vi "MixingGUI_ManyMixtures_OLD.vi"() -> ()   [LabVIEW 2016]
uses:
  <vilib>/Utility/miscctls.llb/LVStringsAndValuesArrayTypeDef.ctl
  <userlib>/Fluigent/Fluigent MFCS/FluigentMFCS_Full.llb/MFCS_EZ Detect.vi
  <userlib>/Fluigent/Fluigent MFCS/FluigentMFCS_Full.llb/MFCS_EZ Initialization.vi
  <userlib>/Fluigent/Fluigent MFCS/FluigentMFCS_Full.llb/MFCS_EZ Write Channel Pressure.vi
  Globals/PressuresGlobal.vi
  Labjack/ValveGlobals.vi
  <vilib>/Utility/file.llb/Write Delimited Spreadsheet (string).vi
  <vilib>/Utility/file.llb/Read Delimited Spreadsheet (string).vi
  <userlib>/_OpenG.lib/array/array.llb/Remove Duplicates from 1D Array (U16)__ogtk.vi
  <vilib>/Utility/xml.llb/Read From XML File(string).vi
  <vilib>/Utility/xml.llb/Write to XML File(string).vi
  <userlib>/Fluigent/Fluigent MFCS/FluigentMFCS_Full.llb/MFCS_EZ Close.vi
  <vilib>/MakerHub/Toolbox/LMH-Toolbox.lvlib
panel:
  out "Set Pressure Cluster":T1={"Control Pressure"=291.6495768427234, "Set Water Mix Pressures"=[nan, nan, nan, nan, nan, 1003.8886388678504, 1033.3198159146239, nan, 1065.755981313159], "Set Odor Pressures"=[nan, nan, 914.431476155127, 919.4749175766236]}
  out "Possible Water Mix Ratios":dbl[](array[numeric])=[0.1, 0.2, 0.30000000000000004, 0.4, 0.5, 0.6, 0.7, 0.7999999999999999, 0.8999999999999999]
  in  "Begin Experiment":bool
  out "Log Folder":path=path "E:/maggot images/Jacob/20180701"
  in  "Master Timing":dbl[][](array[numeric])=[[10.0, 10.0, 10.0], [10.0, 10.0, 10.0]]
  in  "Number of Periods":u16=3
  in  "Master Mix Cluster":T2(array[cluster])=[{"Edit Mixture"=FALSE, "Mixture List"="1.0E-6 1-pentanol", "Odor Time"=10.0, "Water Time"=10.0, "Number of Odors"=1}, {"Edit Mixture"=FALSE, "Mixture List"="1.0E-6 1-pentanol", "Odor Time"=10.0, "Water Time"=10.0, "Number of Odors"=1}, {"Edit Mixture"=FALSE, "Mixture List"="", "Odor Time"=10.0, "Water Time"=10.0, "Number of Odors"=0}, {"Edit Mixture"=FALSE, "Mixture List"="1.0E-7 2,5-dimethylthiazole", "Odor Time"=10.0, "Water Time"=10.0, "Number of Odors"=1}, {"Edit Mixture"=FALSE, "Mixture List"="1.0E-6 acetal", "Odor Time"=10.0, "Water Time"=10.0, "Number of Odors"=1}, {"Edit Mixture"=FALSE, "Mixture List"="1.0E-6 2-phenyl ethanol", "Odor Time"=10.0, "Water Time"=10.0, "Number of Odors"=1}, {"Edit Mixture"=FALSE, "Mixture List"="1.0E-7 2-methoxyphenyl acetate", "Odor Time"=10.0, "Water Time"=10.0, "Number of Odors"=1}, {"Edit Mixture"=FALSE, "Mixture List"="1.0E-7 4-methyl-5-vinythiazole", "Odor Time"=10.0, "Water Time"=10.0, "Number of Odors"=1}, {"Edit Mixture"=FALSE, "Mixture List"="1.0E-6 1-pentanol", "Odor Time"=10.0, "Water Time"=10.0, "Number of Odors"=1}, {"Edit Mixture"=FALSE, "Mixture List"="1.0E-6 1-pentanol\r1.0E-7 4-methyl-5-vinythiazole", "Odor Time"=10.0, "Water Time"=10.0, "Number of Odors"=2}, {"Edit Mixture"=FALSE, "Mixture List"="", "Odor Time"=10.0, "Water Time"=10.0, "Number of Odors"=0}, {"Edit Mixture"=FALSE, "Mixture List"="", "Odor Time"=10.0, "Water Time"=10.0, "Number of Odors"=0}, {"Edit Mixture"=FALSE, "Mixture List"="", "Odor Time"=10.0, "Water Time"=8.0, "Number of Odors"=0}, {"Edit Mixture"=FALSE, "Mixture List"="", "Odor Time"=10.0, "Water Time"=10.0, "Number of Odors"=0}, {"Edit Mixture"=FALSE, "Mixture List"="", "Odor Time"=10.0, "Water Time"=10.0, "Number of Odors"=0}, {"Edit Mixture"=FALSE, "Mixture List"="", "Odor Time"=10.0, "Water Time"=10.0, "Number of Odors"=0}, {"Edit Mixture"=FALSE, "Mixture List"="", "Odor Time"=10.0, "Water Time"=10.0, "Number of Odors"=0}, {"Edit Mixture"=FALSE, "Mixture List"="", "Odor Time"=10.0, "Water Time"=10.0, "Number of Odors"=0}]
  out "Odor Strings":string[](array[string])=["1-pentanol", "3-pentanol", "3-octanol", "2,5-dimethylthiazole", "acetal", "2-phenyl ethanol", "2-methoxyphenyl acetate", "4-methyl-5-vinythiazole"]
  out "Concentration Strings":string[](array[string])=["1.0E-6", "1.0E-7", "1.0E-7", "1.0E-7", "1.0E-6", "1.0E-6", "1.0E-7", "1.0E-7"]
  out "Master Mix Sequence Array":bool[][](array[boolean])=[[TRUE, FALSE, FALSE, FALSE, FALSE, FALSE, FALSE, FALSE], [TRUE, TRUE, TRUE, FALSE, FALSE, FALSE, FALSE, FALSE], [TRUE, FALSE, TRUE, TRUE, FALSE, TRUE, FALSE, FALSE]]
  out "Mix Sequence Array":bool[][](array[boolean])=[[TRUE, FALSE, FALSE, FALSE, FALSE, FALSE, FALSE, FALSE], [TRUE, TRUE, TRUE, FALSE, FALSE, FALSE, FALSE, FALSE], [TRUE, FALSE, TRUE, TRUE, FALSE, TRUE, FALSE, FALSE]]
  out "Calibration Refs":T3={"Pressure Controller List"=[2, 2, 2, 3, 4], "Ratio List"=[0.9, 0.7, 0.6, 0.1, 0.1], "Valve List"=[12, 12, 12, 0, 8]}
  out "Master Pressure Groups":u8[](array[numeric])=[2, 2, 2, 2, 3, 3, 2, 2, 2, 2]
  in  "Master Valves":u16(ring) items=["A1", "A2", "A3", "A4", "B1", "B2", "B3", "B4", "B5", "B6", "B7", "B8", "A5"]
  in  "Tab Control":T4(tab)
  in  "New Animal":bool
  in  "Log File Name":string="MultMixFlowTest"
  in  "Base Folder":path=path "E:/maggot images/Jacob"
  out "load status":string="20180105_config.xml"
  out "status":bool
  in  "Load Button":bool
  in  "Save Button":bool
  in  "Ctr Water Valve":u16(ring)=15 items=["A1", "A2", "A3", "A4", "B1", "B2", "B3", "B4", "B5", "B6", "B7", "B8", "A5", "A6", "A7", "A8"]
  in  "Mix Cluster":T2(array[cluster])=[{"Edit Mixture"=FALSE, "Mixture List"="1.0E-6 1-pentanol", "Odor Time"=10.0, "Water Time"=10.0, "Number of Odors"=1}, {"Edit Mixture"=FALSE, "Mixture List"="1.0E-6 1-pentanol\r1.0E-7 3-pentanol\r1.0E-7 3-octanol", "Odor Time"=10.0, "Water Time"=10.0, "Number of Odors"=3}, {"Edit Mixture"=FALSE, "Mixture List"="1.0E-6 1-pentanol\r1.0E-7 3-octanol\r1.0E-7 2,5-dimethylthiazole\r1.0E-6 2-phenyl ethanol", "Odor Time"=10.0, "Water Time"=10.0, "Number of Odors"=4}]
  in  "Max Number of\nOdors in Mixture":u16=10
  out "Base Dilution":dbl=0.1
  in  "Use Control":bool
  in  "Reset All Calibrations":bool
  in  "Save Odor Inf File":bool
  in  "_run":i16=107
  in  "Sync Camera Acquisition":bool
  out "Saved Log File Name":path
  in  "Set to default pressure":bool
  in  "Mix Water Valve":u16(ring)=12 items=["A1", "A2", "A3", "A4", "B1", "B2", "B3", "B4", "B5", "B6", "B7", "B8", "A5", "A6", "A7", "A8"]
  in  "Ctr Pressure\n Group":u8=1
  in  "Water Mix \nPressure Group":u8=2
  in  "Close All Valves":bool
  in  "Odor":u16[](array[ring])=[0, 1, 2, 3, 4, 5, 6, 7] items=["1-pentanol", "3-pentanol", "3-octanol", "2,5-dimethylthiazole", "acetal", "2-phenylethanol", "2-methoxyphenyl acetate", "4-methyl-5-vinythiazole", "geranyl acetate", "anisole", "water", "methyl phenyl sulfide", "4-methyl-5-vinythiazole", "2,5-dimethylpyrazine", "Fructose", "4-phenyl-2-butanol", "methyl salicylate", "2-heptanone", "menthol", "ethyl acetate", "Fructose", "4-hexen-3-one", "pentyl acetate", "3-octanol", "hexyl acetate", "Add new..."]
  in  "Concentration":u16[](array[ring])=[0, 1, 1, 1, 0, 0, 1, 1] items=["10^-5", "10^-6", "10^-4", "200", "10^-7", "10^-8", "Add new..."]
  in  "Odor Inf Path":path=path "C:/Users/Public/Documents/National Instruments/Fluigent/OdorInf/Data/OdorInfFiles/JB_20171127.txt"
  in  "Append Changes To Odor Inf File":bool=TRUE
  in  "Valves":u16[](array[ring])=[0, 1, 2, 3, 8, 9, 10, 11] items=["A1", "A2", "A3", "A4", "B1", "B2", "B3", "B4", "B5", "B6", "B7", "B8"]
  in  "Pressure Group":enum16{"1", "2", "3", "4"}[](array[ring])=[enum."3", enum."3", enum."3", enum."3", enum."4", enum."4", enum."3", enum."3"]
  in  "Start Water":dbl=10.0
  out "Experiment Time (Sec)":dbl=70.0
  in  "Calibrate Pressures":bool
  out "Duplicates!":bool
  in  "Zero Pressure":bool
  in  "Ctr Odor Valve":u16(ring)=14 items=["A1", "A2", "A3", "A4", "B1", "B2", "B3", "B4", "B5", "B6", "B7", "B8", "A5", "A6", "A7", "A8"]
  in  "Calibration Mode":T5(ring)
  in  "Refill!":bool[](array[boolean])=[FALSE, FALSE, FALSE, FALSE, FALSE, FALSE, FALSE, FALSE, FALSE, FALSE, FALSE, FALSE, FALSE]
  out "Odor \nLevel":T6 {"Tank 13" scale=0.0..10.0; "Tank 12" scale=0.0..10.0; "Tank 11" scale=0.0..10.0; "Tank 10" scale=0.0..10.0; "Tank 9" scale=0.0..10.0; "Tank 8" scale=0.0..10.0; "Tank 7" scale=0.0..10.0; "Tank 6" scale=0.0..10.0; "Tank 5" scale=0.0..10.0; "Tank 4" scale=0.0..10.0; "Tank 3" scale=0.0..10.0; "Tank 2" scale=0.0..10.0; "Tank" scale=0.0..10.0}
  in  "stop":bool=TRUE
  in  "Start\nWater 2":dbl=10.0
  in  "Timing":dbl[][](array[numeric])=[[10.0, 10.0, 10.0], [10.0, 10.0, 10.0]]
  out "Odor List":string[](array[string])=["1.0E-6 1-pentanol", "1.0E-7 3-pentanol", "1.0E-7 3-octanol", "1.0E-7 2,5-dimethylthiazole", "1.0E-6 acetal", "1.0E-6 2-phenyl ethanol", "1.0E-7 2-methoxyphenyl acetate", "1.0E-7 4-methyl-5-vinythiazole"]
  in  "Mix Sequence Control":bool[][](array[boolean])=[[TRUE, TRUE, TRUE], [FALSE, TRUE, FALSE], [FALSE, TRUE, TRUE], [FALSE, FALSE, TRUE], [FALSE, FALSE, FALSE], [FALSE, FALSE, TRUE], [FALSE, FALSE, FALSE], [FALSE, FALSE, FALSE]]
  in  "Set to default pressure 2":bool
  in  "Zero Pressure 2":bool
  in  "Show Flow VI":bool
  in  "Flow 1 Filter Time":dbl=0.2
  in  "Flow 2 Filter Time":dbl=5.0
  in  "Mix Water Pressure Channel":u16=2
  in  "Control Pressure Channel":u16=1
  out "Current Pressure":dbl[](array[numeric])=[291.6055908203125, 1003.57763671875, 915.2123413085938, 918.9993896484375]
  in  "Manual Set Pressures":dbl[](array[numeric])=[291.6495768427234, 1037.0302734375, 914.431476155127, 914.431476155127]
  in  "Total Odor Flow":dbl=425.0
  in  "Total Flow Setpoint":dbl=531.25
  out "Flow Meter 1 (water flow)":cluster{"[0]":dbl}(graph)={"[0]"=265.3103448275862}
  out "Flow Meter 2 (total flow)":cluster{"[0]":dbl}(graph)={"[0]"=529.7241379310345}
  in  "Values to Display":dbl=2000.0
  out "Default Pressures":dbl[](array[numeric])=[291.6495768427234, 1037.0302734375, 914.431476155127, 914.431476155127]
  out "Current Flow Rates":dbl[](array[numeric])=[265.3103448275862, 529.7241379310345]
  out "Master Valves":T7=[{"String"="A1", "Value"=0.0}, {"String"="A2", "Value"=1.0}, {"String"="A3", "Value"=2.0}, {"String"="A4", "Value"=3.0}, {"String"="B1", "Value"=4.0}, {"String"="B2", "Value"=5.0}, {"String"="B3", "Value"=6.0}, {"String"="B4", "Value"=7.0}, {"String"="B5", "Value"=8.0}, {"String"="B6", "Value"=9.0}, {"String"="B7", "Value"=10.0}, {"String"="B8", "Value"=11.0}, {"String"="A5", "Value"=12.0}]
  # "Odor\nTime"
  # "Water\nTime"
  # "Number of Odors"
  # "Mixture"
  # "log_"
  # ".txt"
  # "Odor Time"
  # "Water Time"
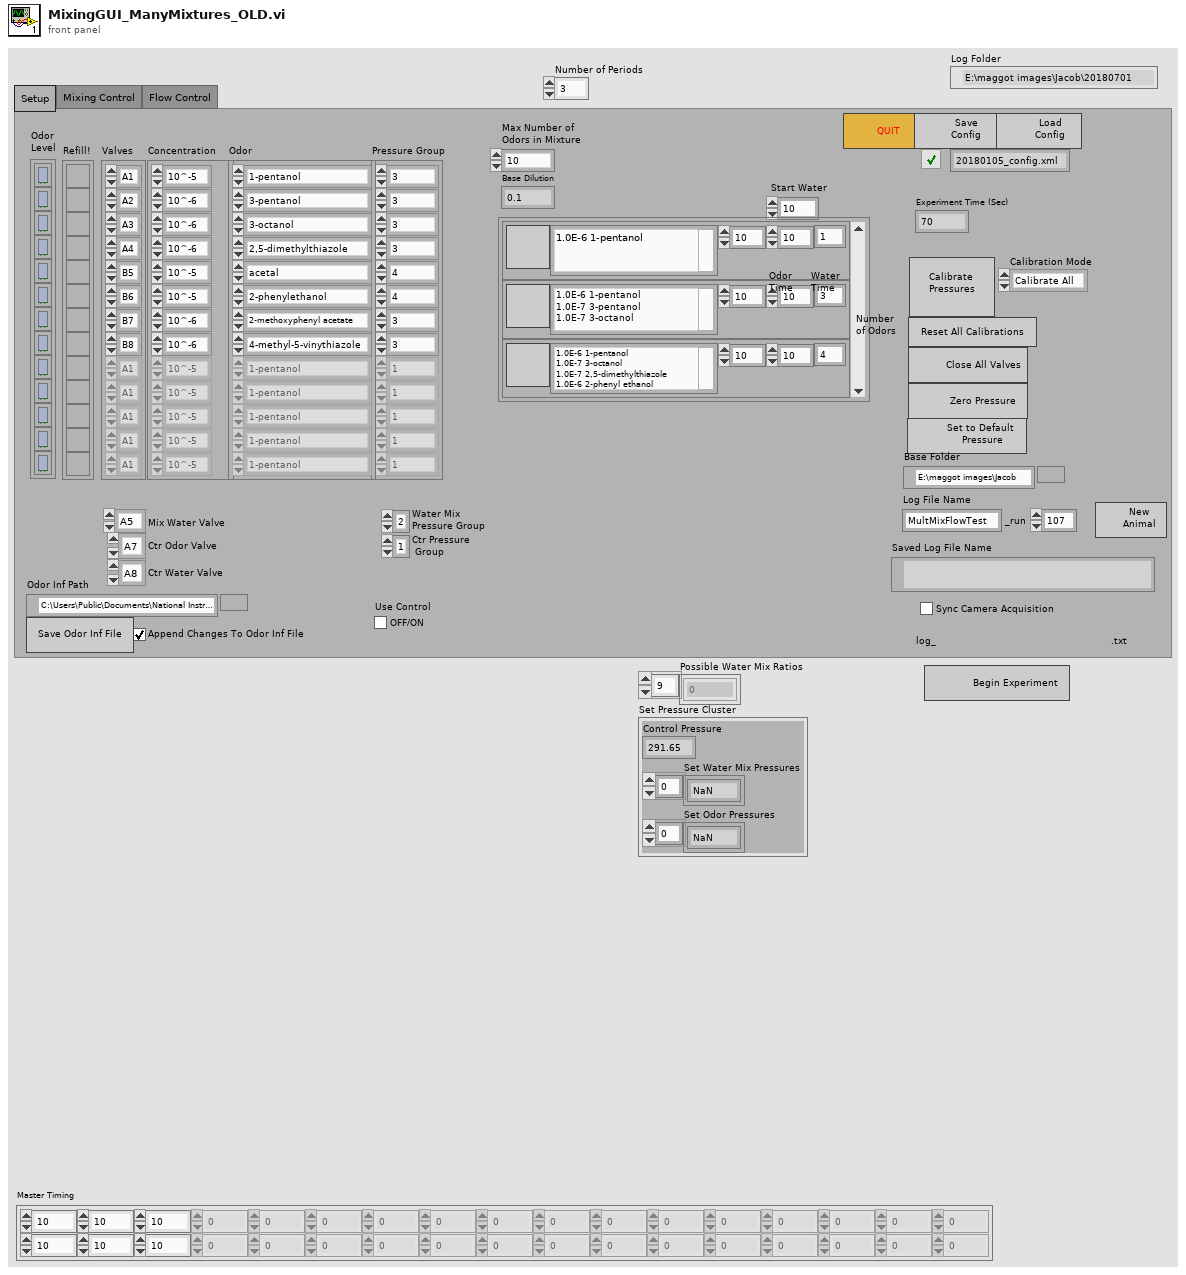
[diagram p1: front panel]
types:
  T1 = cluster{"Control Pressure":dbl, "Set Water Mix Pressures":dbl[], "Set Odor Pressures":dbl[]}
  T2 = cluster{"Edit Mixture":bool, "Mixture List":string, "Odor Time":dbl, "Water Time":dbl, "Number of Odors":u16}[]
  T3 = cluster{"Pressure Controller List":u8[], "Ratio List":dbl[], "Valve List":u16[]}
  T4 = enum32{"Setup", "Mixing Control", "Flow Control"}
  T5 = enum16{"Calibrate All", "Control Only", "Odors Only"}
  T6 = cluster{"Tank":dbl, "Tank 2":dbl, "Tank 3":dbl, "Tank 4":dbl, "Tank 5":dbl, "Tank 6":dbl, "Tank 7":dbl, "Tank 8":dbl, "Tank 9":dbl, "Tank 10":dbl, "Tank 11":dbl, "Tank 12":dbl, "Tank 13":dbl}
  T7 = typedef "LVStringsAndValuesArrayTypeDef.ctl" = cluster{"String":string, "Value":ext}[]
  T8 = enum32{"Invalid", "Standard", "Closed", "Hidden", "Minimized", "Maximized"}
  T9 = cluster{"Ctr Odor Valve":u16, "Water Mix Valve":u16, "Total Odor Flow":dbl, "Total Flow Setpoint":dbl, "Control Pressure Channel":u16, "Mix Water Pressure Channel":u16}
  T10 = typedef "_EZmfcsSN.ctl" = u16
  T11 = typedef "_EZmfcsRefNum.ctl" = refnum<k1>
  T12 = enum32{"Invalid", "Standard", "Closed", "Hidden", "Minimized", "Maximized"}[]
  T13 = cluster{"[0]":dbl, "[1]":dbl, "[2]":dbl, "[3]":dbl, "[4]":dbl, "[5]":dbl, "[6]":dbl, "[7]":dbl, "[8]":dbl, "[9]":dbl, "[10]":dbl, "[11]":dbl, "[12]":dbl}
  T14 = cluster{"Edit Mixture":bool, "Mixture List":string, "Odor Time":dbl, "Water Time":dbl, "Number of Odors":u16}
  T15 = cluster{"Odor Names":string[], "Concentration Names":string[], "Mix Sequence Array":bool[][], "Sequence Time":dbl[]}
  T16 = cluster{"Flowboards":enum16{"A", "B", "C"}[], "Channels":enum16{"1", "2", "3", "4", "5", "6", "7", "8"}[], "States":bool[]}[]
  T17 = cluster{"t":dbl[], "Pressures":dbl[][], "Flow Rate":dbl[][]}
  T18 = cluster{"Valves":u16[], "Concentration":u16[], "Odor":u16[], "Pressure Group":enum16{"1", "2", "3", "4"}[], "Mix Sequence Array":bool[][], "Start Water":dbl, "Base Dilution":dbl, "Max Number of\nOdors in Mixture":u16, "Default Pressures":dbl[], "Set Pressure Cluster":cluster{"Control Pressure":dbl, "Set Water Mix Pressures":dbl[], "Set Odor Pressures":dbl[]}, "Mix Cluster":cluster{"Edit Mixture":bool, "Mixture List":string, "Odor Time":dbl, "Water Time":dbl, "Number of Odors":u16}[], "Calibration Refs":cluster{"Pressure Controller List":u8[], "Ratio List":dbl[], "Valve List":u16[]}, "Number of Periods":u16}
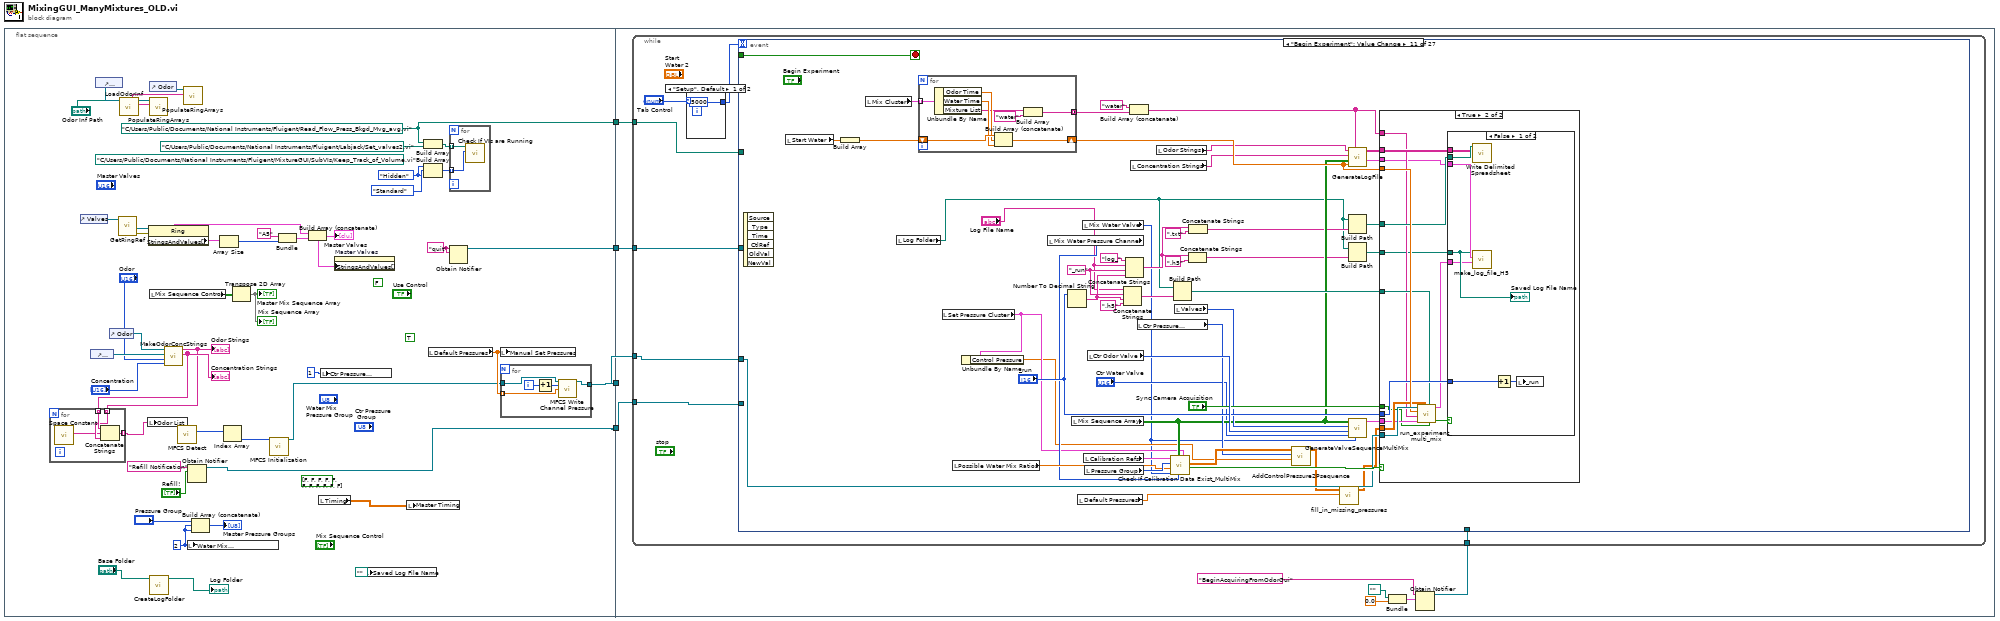
[diagram p0: block diagram]
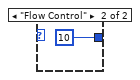
[diagram p2: hidden frame]
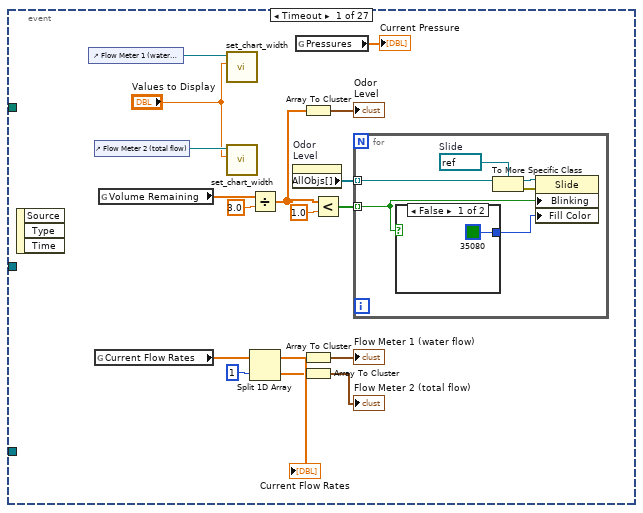
[diagram p3: hidden frame]
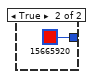
[diagram p4: hidden frame]
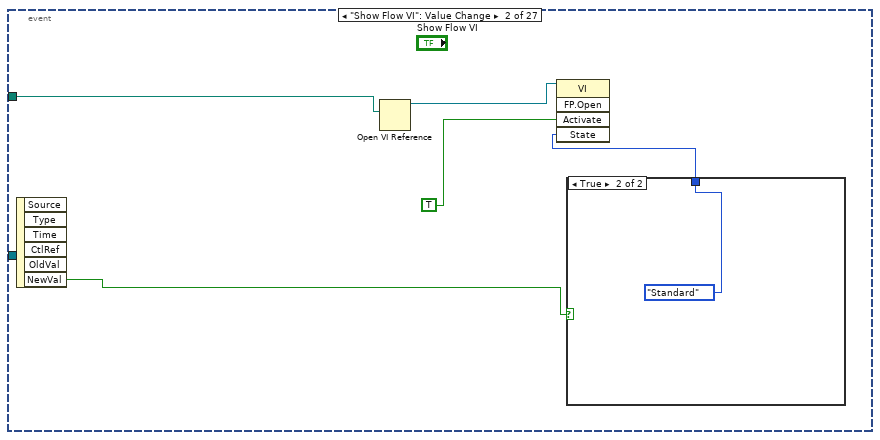
[diagram p5: hidden frame]
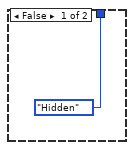
[diagram p6: hidden frame]
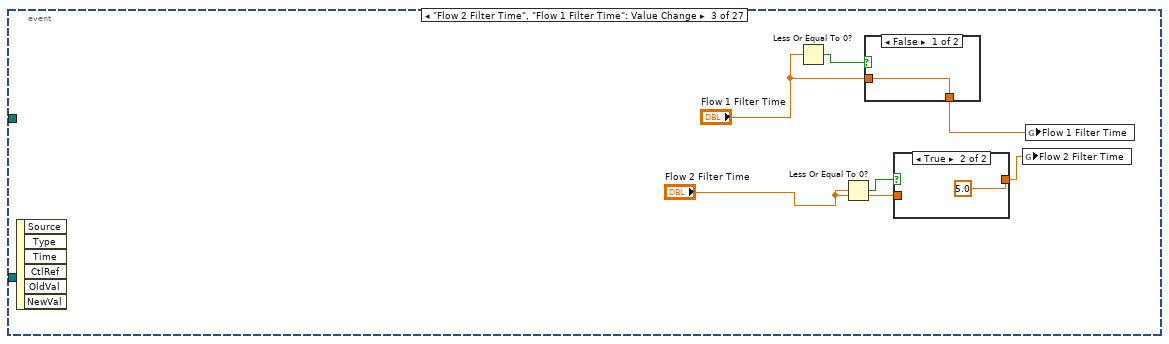
[diagram p7: hidden frame]
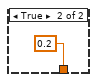
[diagram p9: hidden frame]
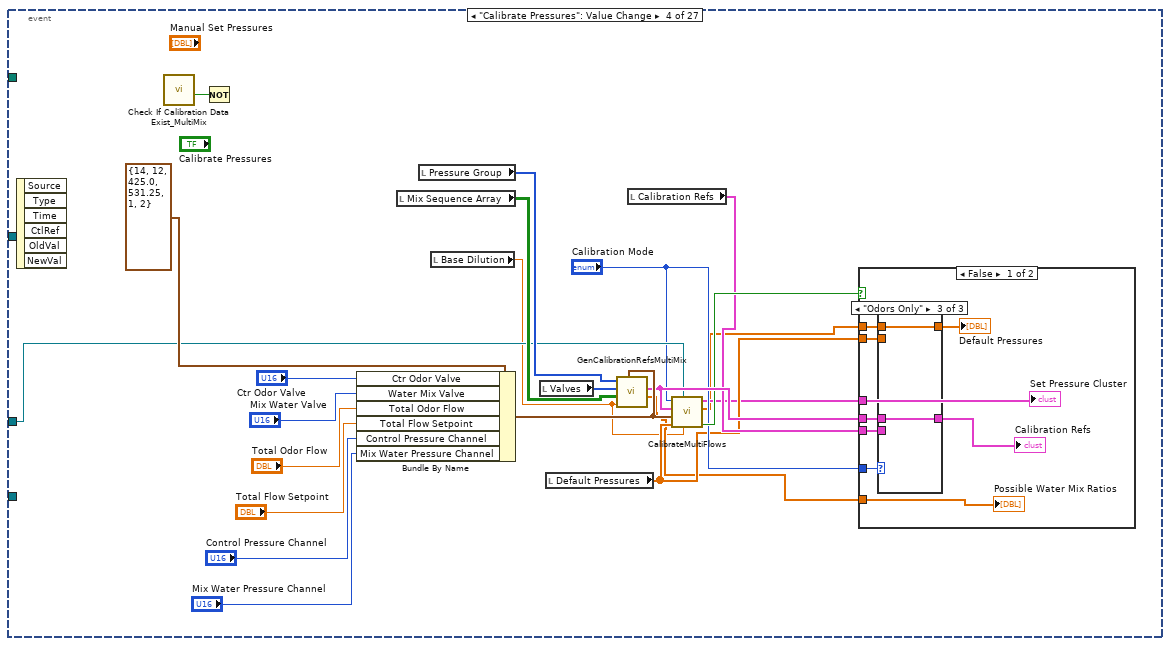
[diagram p10: hidden frame]
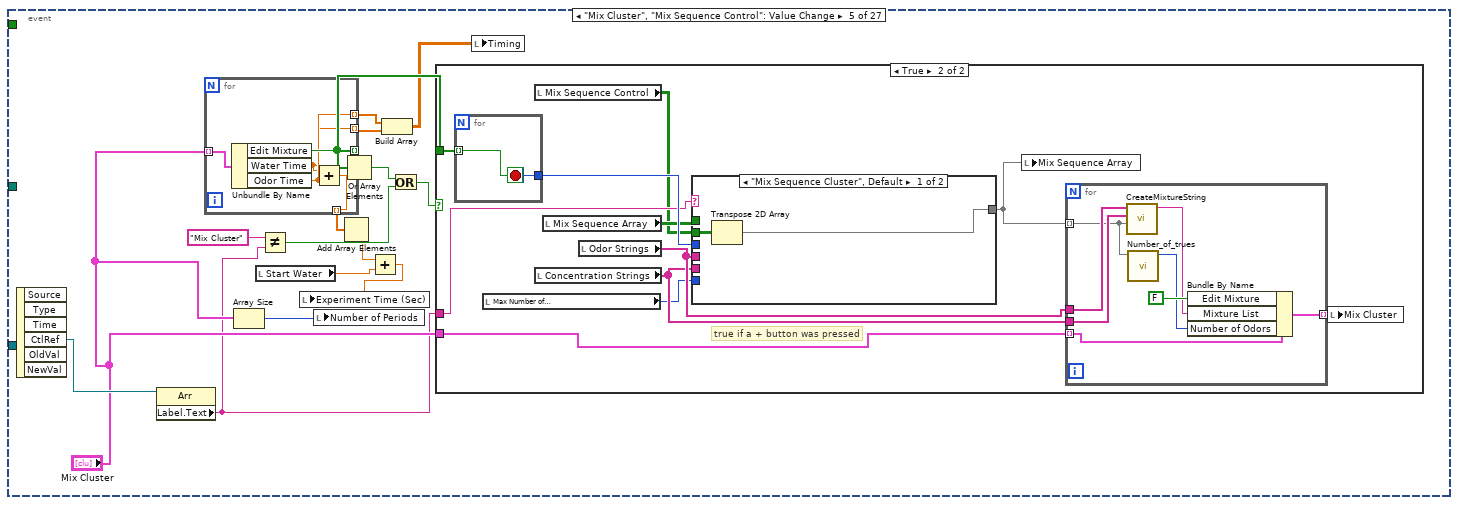
[diagram p14: hidden frame]
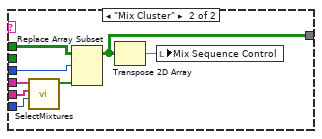
[diagram p16: hidden frame]
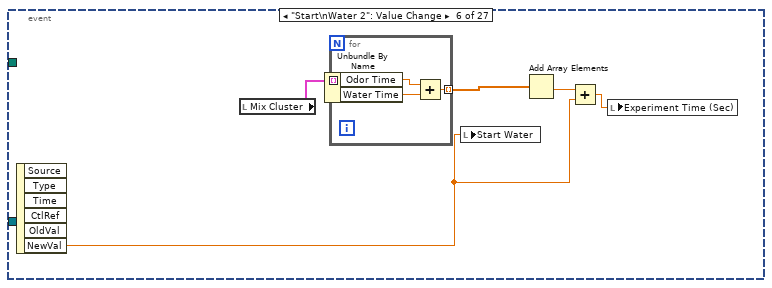
[diagram p17: hidden frame]
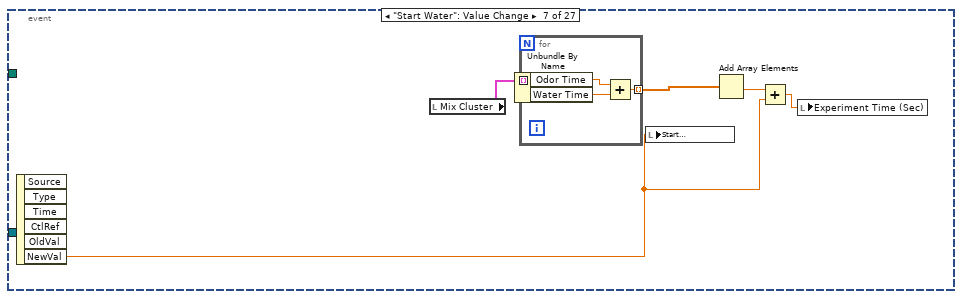
[diagram p18: hidden frame]
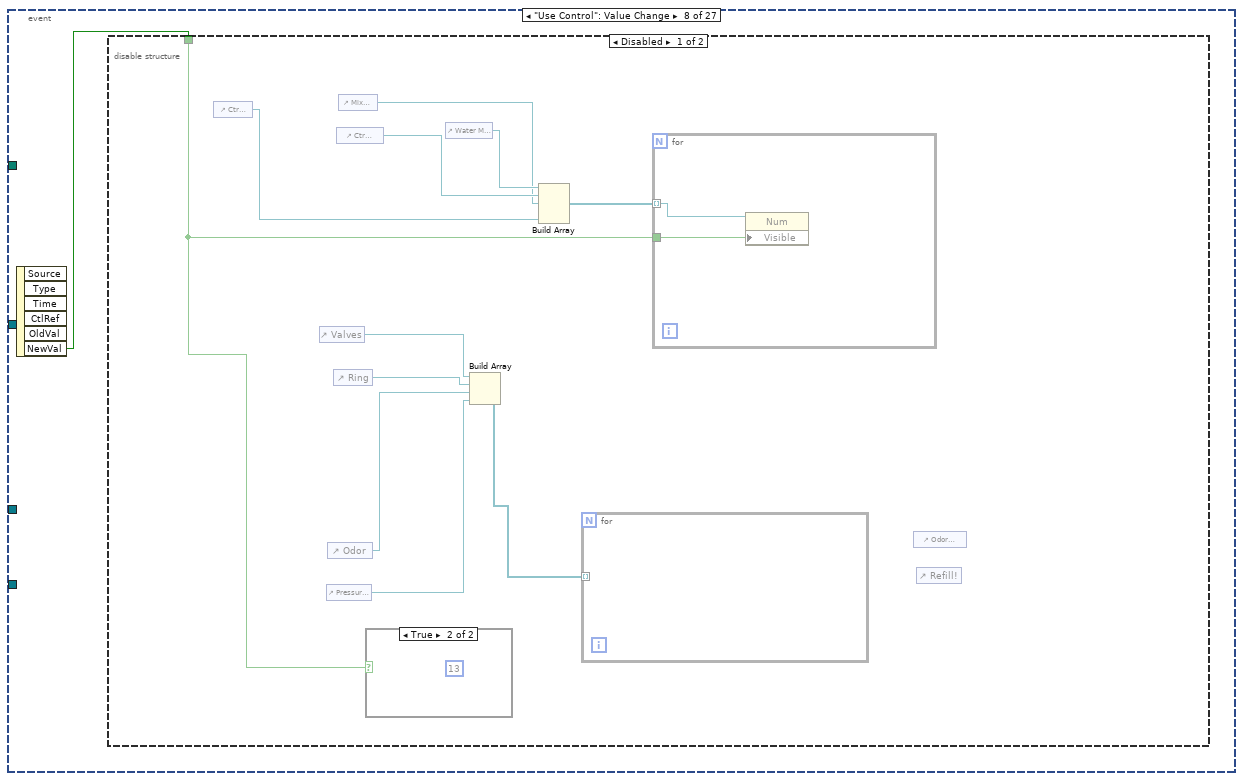
[diagram p19: hidden frame]
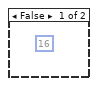
[diagram p20: hidden frame]
diagram:
  n1 = flat-sequence {
    tunnel: [w6] -> w4
    tunnel: [w29] -> w3
    tunnel: [w19] -> w2
    tunnel: [w17] -> w1
    tunnel: w4 -> [w70]
    tunnel: w3 -> [w64]
    tunnel: w2 -> [w63]
    tunnel: w1 -> [w62]
    frame #0 {
      w18 = "quit" ("name (unnamed)")
      (unwired) path "C:/Users/Public/Documents/National Instruments/Fluigent/MixtureGUI/SubVIs/Keep_Track_of_Volume.vi"
      (unwired) bool[] [FALSE, FALSE, FALSE, FALSE, FALSE, FALSE, FALSE, FALSE, FALSE, FALSE, FALSE] ("Refill!")
      (unwired) FALSE ("Visible")
      (unwired) TRUE ("Calibration Required")
      w28 = T8."Hidden" ("State")
      w19 = path "C:/Users/Public/Documents/National Instruments/Fluigent/Read_Flow_Press_Bkgd_Mvg_avg.vi"
      w25 = u8 2 ("Water Mix Pressure Group")
      n2 = control-ref of="Valves"() -> (w46:refnum<vi>)
      n3 = control-ref of="Concentration"() -> (w23:refnum<vi>)
      n4 = control-ref of="Concentration"() -> (w42:refnum<vi>)
      n5 = control-ref of="Odor"() -> (w24:refnum<vi>)
      n6 = call "GetRingRef.vi"("Array Reference"=w46) -> ("error out"=w45:errorcluster, "Ring Reference"=w44:refnum<vi>)  [unwired: 9 in]
      n7 = call "LoadOdorInf.vi"("file path (dialog if empty)"="Odor Inf Path") -> ("Concentration"=w43:string[], "Odor"=w41:string[])  [unwired: 9 in]
      n8 = property class="Ring"(reference=w44, error in=w45) -> ("StringsAndValues[]"=w50:T7)  [unwired: 2 out]
      n9 = control-ref of="Odor"() -> (w40:refnum<vi>)
      n10 = call "PopulateRingArrays.vi"("array"=w43, "Array Reference"=w42) -> ()  [unwired: 8 in, 2 out]
      n11 = local read "Mix Sequence Control"() -> (w9:bool[][])
      n12 = call "CreateLogFolder.vi"("Base Folder"="Base Folder") -> ("Path Out"=→"Log Folder":path)  [unwired: 9 in, 1 out]
      n13 = call "MakeOdorConcStrings.vi"(8:"Concentration"="Concentration", 9:"Odor"="Odor", 10:"Concentration"=w23, 11:"Odor"=w24) -> ("Concentration Strings"=w16:string[], "Odor Strings"=w15:string[])  [unwired: 6 in]
      "Concentration Strings" <- w16
      "Odor Strings" <- w15
      n14 = for {
        tunnel: w16 -> [w59] mode=indexing
        tunnel: w15 -> [w58] mode=indexing
        tunnel: [w56] -> w14 mode=indexing
        n15 = call <vilib>:"Space Constant.vi"() -> ("String"=w57:string)
        n16 = Concatenate Strings(w59, w57, w58) -> (w56:string)
      }
      n17 = local write "Odor List"(w14) -> ()
      n18 = call-poly <userlib>:"MFCS Detect.vi"() -> ("[SN MFCS_EZ]"=w38:T10[])  [unwired: 14 in, 1 out]
      n19 = call "PopulateRingArrays.vi"("array"=w41, "Array Reference"=w40) -> ()  [unwired: 8 in, 2 out]
      n20 = local write "Water Mix \nPressure Group"(w25) -> ()
      n21 = Obtain Notifier(name (unnamed)="Refill Notification", notification data type="Refill!") -> (notifier out=w29:refnum<notifier>)  [unwired: 2 in, 2 out]
      n22 = Build Array (concatenate)("Pressure Group", w25, w25) -> (→"Master Pressure Groups":u16[])
      n23 = Array Size(array=w50) -> (size(s)=w48:i32)
      n24 = Index Array(array=w38) -> (element=w37:T10)  [unwired: 1 in]
      n25 = Transpose 2D Array(2D array=w9) -> (transposed array=→"Mix Sequence Array" →"Master Mix Sequence Array":bool[][])
      n26 = call-poly <userlib>:"MFCS Initialization.vi"("SN MFCS_EZ"=w37) -> ("MFCS_EZ"=w7:T11)  [unwired: 12 in, 2 out]
      n27 = Bundle("A5", w48) -> (w49:cluster{string, i32})  [unwired: 1 in]
      n28 = Build Array (concatenate)(w50, w49) -> (w36:T7)
      "Master Valves" <- w36
      n29 = local read "Timing"() -> (w13:dbl[][])
      n30 = local write "Ctr Pressure\n Group"(u8 1 ("Ctr Pressure Group")) -> ()
      n31 = property on="Master Valves" class="Ring (strict)"("StringsAndValues[]"=w36) -> ()  [unwired: 2 in, 2 out]
      n32 = local write "Saved Log File Name"(path "" ("Log File Name")) -> ()
      n33 = local write "Master Timing"(w13) -> ()
      n34 = Build Array(w19, path "C:/Users/Public/Documents/National Instruments/Fluigent/Labjack/Set_valves2.vi") -> (w33:path[])
      n35 = Build Array(w28, T8."Standard" ("State"), w28) -> (w31:T12)
      n36 = local read "Default Pressures"() -> (w8:dbl[])
      n37 = for {
        tunnel: w33 -> [w61] mode=indexing
        tunnel: w31 -> [w60] mode=indexing
        n38 = call "Check If VIs are Running.vi"("State"=w60, "Path"=w61) -> ()  [unwired: 9 in, 1 out]
      }
      n39 = Obtain Notifier(name (unnamed)=w18, notification data type=w18) -> (notifier out=w17:refnum<notifier>)  [unwired: 2 in, 2 out]
      n40 = local write "Manual Set Pressures"(w8) -> ()
      n41 = for {
        tunnel: w7 -> [w55]
        tunnel: w8 -> [w54] mode=indexing
        tunnel: [w51] -> w6
        i -> [w53]
        n42 = Increment(x=w53) -> (x+1=w52:i32)
        n43 = call-poly <userlib>:"MFCS Write Channel Pressure.vi"("MFCS_EZ"=w55, "Channel Number (default=1)"=w52, "Pressure (mBar)"=w54) -> ("MFCS_EZ out"=w51:T11)  [unwired: 11 in, 1 out]
      }
    }
    frame #1 {
      n44 = Bundle("Log File Name"=path "", 0.0) -> (w66:cluster{"Log File Name":path, dbl})  [unwired: 1 in]
      n45 = Obtain Notifier(name (unnamed)="BeginAcquiringFromOdorGui", notification data type=w66) -> (notifier out=w68:refnum<notifier>)  [unwired: 2 in, 2 out]
      n46 = while {
        tunnel: w70 -> [w75]
        tunnel: w68 -> [w74]
        tunnel: w64 -> [w73]
        tunnel: w63 -> [w72]
        tunnel: w62 -> [w71]
        stop <- w78 stop-if-true
        n47 = case shown="\"Setup\", Default" "Tab Control" {
          tunnel: [5000 10] -> w76
          frame "Setup", Default {
          }
          frame "Flow Control" {
          }
        }
        n48 = event shown="[10] \"Begin Experiment\": Value Change" {
          selector: _ -> [_ _ _ _ _ _ _ _ _ _ _ _ _ _ _ _ _ _ _ _ _ _ _ _ _ _ _]
          dyn-events: _ -> [_ _ _ _ _ _ _ _ _ _ _ _ _ _ _ _ _ _ _ _ _ _ _ _ _ _ _]
          timeout: w76 -> [_ _ _ _ _ _ _ _ _ _ _ _ _ _ _ _ _ _ _ _ _ _ _ _ _ _ _]
          tunnel: [_ _ _ _ _ _ _ _ _ _ _ _ _ _ _ _ _ _ _ _ _ _ _ _ _ _ TRUE] -> w78
          tunnel: w75 -> [_ _ _ w130 _ _ _ _ _ _ w291 _ _ w348 _ w354 _ _ w368 _ _ _ _ _ _ _ w624]
          tunnel: w74 -> [_ _ _ _ _ _ _ _ _ _ _ _ _ _ _ _ _ _ _ _ _ _ _ _ _ _ _]
          tunnel: w73 -> [_ _ _ _ _ _ _ _ _ w247 _ _ _ _ _ _ _ _ _ _ _ _ _ _ _ _ _]
          tunnel: w72 -> [_ w110 _ _ _ _ _ _ _ _ _ _ _ _ _ _ _ _ _ _ _ _ _ _ _ _ _]
          tunnel: w71 -> [_ _ _ _ _ _ _ _ _ _ _ _ _ _ _ _ _ _ _ _ _ _ _ _ _ _ w621]
          event Timeout {
            n49 = event-data() -> ()  [unwired: 1 in, 3 out]
            n50 = control-ref of="Flow Meter 1 (water flow)"() -> (w90:refnum<vi>)
            n51 = control-ref of="Flow Meter 2 (total flow)"() -> (w89:refnum<vi>)
            n52 = global read "PressuresGlobal.vi" "Current Flow Rates"() -> (w94:dbl[])
            "Current Flow Rates" <- w94
            n53 = global read "ValveGlobals.vi" "Volume Remaining"() -> (w82:dbl[])
            n54 = call "set_chart_width.vi"("Values to Display"="Values to Display", "Ctl Refnum"=w90) -> ()  [unwired: 10 in]
            n55 = call "set_chart_width.vi"("Values to Display"="Values to Display", "Ctl Refnum"=w89) -> ()  [unwired: 10 in]
            n56 = Divide(x=w82, y=3.0) -> (x/y=w81:dbl[])
            n57 = Split 1D Array(array=w94, index=1) -> (first subarray=w92:dbl[], second subarray=w91:dbl[])
            n58 = property on="Odor \nLevel" class="Clust (strict)"() -> ("AllObjs[]"=w85:refnum<vi>[])  [unwired: 2 in, 2 out]
            n59 = global read "PressuresGlobal.vi" "Pressures"() -> (→"Current Pressure":dbl[])
            n60 = Array To Cluster(array=w81) -> (cluster=→"Odor \nLevel":T13)
            n61 = Array To Cluster(array=w92) -> (cluster=→"Flow Meter 1 (water flow)":cluster{"[0]":dbl})
            n62 = Array To Cluster(array=w91) -> (cluster=→"Flow Meter 2 (total flow)":cluster{"[0]":dbl})
            n63 = Less?(x=w81, y=1.0) -> (x < y?=w86:bool[])
            n64 = for {
              tunnel: w86 -> [w99] mode=indexing
              tunnel: w85 -> [w103] mode=indexing
              w102 = refnum<vi> refnum  # Slide
              n65 = case shown="False" w99 {
                tunnel: [u32 35080 u32 15665920] -> w98
                frame False {
                }
                frame True {
                }
              }
              n66 = To More Specific Class(target class=w102, reference=w103) -> (specific class reference=w101:refnum<vi>, error out=w100:errorcluster)  [unwired: 1 in]
              n67 = property class="Slide"(reference=w101, error in=w100, "Blinking"=w99, "Fill Color"=w98) -> ()  [unwired: 2 out]
            }
          }
          event "Show Flow VI": Value Change {
            n68 = event-data() -> ("NewVal"=w108:bool)  [unwired: 1 in, 5 out]
            n69 = Open VI Reference(vi path=w110) -> (vi reference=w109:refnum<vi>)  [unwired: 5 in, 1 out]
            n70 = case shown="True" w108 {
              tunnel: [T8."Hidden" ("State") T8."Standard" ("State")] -> w106
              frame False {
              }
              frame True {
              }
            }
            n71 = invoke class="VI" method="FP.Open"(reference=w109, "Activate"=TRUE ("Activate?"), "State"=w106) -> ()  [unwired: 2 in, 5 out]
          }
          event "Flow 2 Filter Time", "Flow 1 Filter Time": Value Change {
            n72 = event-data() -> ()  [unwired: 1 in, 6 out]
            n73 = Less Or Equal To 0?(x="Flow 1 Filter Time") -> (x <= 0?=w118:bool)
            n74 = Less Or Equal To 0?(x="Flow 2 Filter Time") -> (x <= 0?=w115:bool)
            n75 = case shown="False" w118 {
              tunnel: [w121 0.2 ("Flow 1 Filter Time")] -> w117
              tunnel: "Flow 1 Filter Time" -> [w121 _]
              frame False {
              }
              frame True {
              }
            }
            n76 = case shown="True" w115 {
              tunnel: [w119 5.0 ("Flow 1 Filter Time")] -> w113
              tunnel: "Flow 2 Filter Time" -> [w119 _]
              frame False {
              }
              frame True {
              }
            }
            n77 = global write "PressuresGlobal.vi" "Flow 2 Filter Time"(w113) -> ()
            n78 = global write "PressuresGlobal.vi" "Flow 1 Filter Time"(w117) -> ()
          }
          event "Calibrate Pressures": Value Change {
            n79 = event-data() -> ()  [unwired: 1 in, 6 out]
            n80 = call "Check If Calibration Data Exist_MultiMix.vi"() -> ("Calibration Data Exists?"=w137:bool)  [unwired: 10 in, 1 out]
            n81 = Not(x=w137) -> ()  [unwired: 1 out]
            n82 = Bundle By Name(cluster=T9 {"Ctr Odor Valve"=14, "Water Mix Valve"=12, "Total Odor Flow"=425.0, "Total Flow Setpoint"=531.25, "Control Pressure Channel"=1, "Mix Water Pressure Channel"=2} ("Misselaneous Parameters"), "Ctr Odor Valve"="Ctr Odor Valve", "Water Mix Valve"="Mix Water Valve", "Total Odor Flow"="Total Odor Flow", "Total Flow Setpoint"="Total Flow Setpoint", "Control Pressure Channel"="Control Pressure Channel", "Mix Water Pressure Channel"="Mix Water Pressure Channel") -> (w133:T9)
            n83 = local read "Mix Sequence Array"() -> (w136:bool[][])
            n84 = local read "Pressure Group"() -> (w134:enum16{"1", "2", "3", "4"}[])
            n85 = local read "Base Dilution"() -> (w123:dbl)
            n86 = local read "Valves"() -> (w135:u16[])
            n87 = local read "Default Pressures"() -> (w127:dbl[])
            n88 = call "GenCalibrationRefsMultiMix.vi"("Misselaneous Parems"=w133, "Base Dilution"=w123, "Mix Sequence Array"=w136, "Valves"=w135, "Pressure Group"=w134) -> ("Possible Water Mix Ratios"=w126:dbl[], "Calibration Refs"=w132:T3)  [unwired: 5 in]
            n89 = local read "Calibration Refs"() -> (w128:T3)
            n90 = call "CalibrateMultiFlows.vi"("Base Dilution"=w123, "MFCS_EZ"=w130, "Manual Default Set Pressures"=w127, "Missaleneouns Parems"=w133, "Calibration Refs"=w132, "Calibration Mode"="Calibration Mode") -> ("Aborted?"=w131:bool, "New Manual Pressure"=w124:dbl[], "Set Pressure Cluster"=w125:T1)  [unwired: 3 in]
            n91 = case shown="False" w131 {
              tunnel: w132 -> [w152 _]
              tunnel: "Calibration Mode" -> [w153 _]
              tunnel: w128 -> [w149 _]
              tunnel: w127 -> [w148 _]
              tunnel: w126 -> [w147 _]
              tunnel: w125 -> [w145 _]
              tunnel: w124 -> [w146 _]
              frame False {
                n92 = case shown="\"Odors Only\"" w153 {
                  tunnel: w152 -> [w155 _ w159]
                  tunnel: [w155 w157 w159] -> w151
                  tunnel: [w154 w156 w158] -> w150
                  tunnel: w149 -> [_ w157 _]
                  tunnel: w148 -> [_ w156 _]
                  tunnel: w146 -> [w154 _ w158]
                  frame "Calibrate All", Default {
                  }
                  frame "Control Only" {
                  }
                  frame "Odors Only" {
                  }
                }
                "Calibration Refs" <- w151
                "Default Pressures" <- w150
                "Possible Water Mix Ratios" <- w147
                "Set Pressure Cluster" <- w145
              }
              frame True {
              }
            }
          }
          event "Mix Cluster", "Mix Sequence Control": Value Change {
            n93 = event-data() -> ("CtlRef"=w173:refnum<vi>)  [unwired: 1 in, 5 out]
            n94 = property class="Arr"(reference=w173) -> ("Label.Text"=w171:string)  [unwired: 1 in, 2 out]
            n95 = for {
              tunnel: "Mix Cluster" -> [w211] mode=indexing
              tunnel: [w210] -> w175 mode=indexing
              tunnel: [w209] -> w166 mode=indexing
              tunnel: [w208] -> w162 mode=indexing
              tunnel: [w207] -> w161 mode=indexing
              n96 = Unbundle By Name(w211) -> ("Edit Mixture"=w210:bool, "Water Time"=w207:dbl, "Odor Time"=w208:dbl)
              n97 = Add(x=w207, y=w208) -> (x+y=w209:dbl)
            }
            n98 = Array Size(array="Mix Cluster") -> (size(s)=w174:i32)
            n99 = local read "Start Water"() -> (w165:dbl)
            n100 = Not Equal?(x="Mix Cluster", y=w171) -> (x != y?=w168:bool)
            n101 = local write "Number of Periods"(w174) -> ()
            n102 = Add Array Elements(numeric array=w166) -> (sum=w164:dbl)
            n103 = Or Array Elements(Boolean array=w175) -> (logical OR=w169:bool)
            n104 = Add(x=w164, y=w165) -> (x+y=w163:dbl)
            n105 = local write "Experiment Time (Sec)"(w163) -> ()
            n106 = Build Array(w162, w161) -> (w160:dbl[][])
            n107 = Or(x=w169, y=w168) -> (x .or. y?=w167:bool)
            n108 = case shown="True" w167 {
              tunnel: w175 -> [_ w185]
              tunnel: "Mix Cluster" -> [_ w178]
              tunnel: w171 -> [_ w180]
              frame False {
              }
              frame True {
                # "true if a + button was pressed"
                n109 = for {
                  tunnel: [w188] -> w186
                  tunnel: w185 -> [w187] mode=indexing
                  i -> [w188]
                  stop <- w187 stop-if-true
                }
                n110 = local read "Max Number of\nOdors in Mixture"() -> (w182:u16)
                n111 = local read "Mix Sequence Control"() -> (w179:bool[][])
                n112 = local read "Concentration Strings"() -> (w183:string[])
                n113 = local read "Mix Sequence Array"() -> (w181:bool[][])
                n114 = local read "Odor Strings"() -> (w184:string[])
                n115 = case shown="\"Mix Sequence Cluster\", Default" w180 {
                  tunnel: w186 -> [_ w206]
                  tunnel: w184 -> [_ w205]
                  tunnel: w183 -> [_ w204]
                  tunnel: w182 -> [_ w203]
                  tunnel: w181 -> [_ w202]
                  tunnel: [w197 w200] -> w176
                  tunnel: w179 -> [w198 _]
                  frame "Mix Sequence Cluster", Default {
                    n116 = Transpose 2D Array(2D array=w198) -> (transposed array=w197:bool[][])
                  }
                  frame "Mix Cluster" {
                    n117 = call "SelectMixtures.vi"("Max Number of Odors"=w203, "Concentrations"=w204, "Odors"=w205) -> ("Odor Mixtures"=w201:bool[])  [unwired: 6 in, 1 out]
                    n118 = Replace Array Subset(array=w202, new element=w201, index (row)=w206) -> (w200:bool[][])  [unwired: 1 in]
                    n119 = Transpose 2D Array(2D array=w200) -> (transposed array=w199:bool[][])
                    n120 = local write "Mix Sequence Control"(w199) -> ()
                  }
                }
                n121 = local write "Mix Sequence Array"(w176) -> ()
                n122 = for {
                  tunnel: w184 -> [w196]
                  tunnel: w183 -> [w195]
                  tunnel: w178 -> [w194] mode=indexing
                  tunnel: [w189] -> w177 mode=indexing
                  tunnel: w176 -> [w190] mode=indexing
                  n123 = call "CreateMixtureString.vi"("Odor Mixtures"=w190, "Concentrations"=w195, "Odors"=w196) -> ("Odor Mixture String"=w192:string)  [unwired: 8 in]
                  n124 = call "Number_of_trues.vi"("Boolean Array"=w190) -> ("Number of True Values"=w191:i32)  [unwired: 10 in]
                  n125 = Bundle By Name(cluster=w194, "Edit Mixture"=FALSE, "Mixture List"=w192, "Number of Odors"=w191) -> (w189:T14)
                }
                n126 = local write "Mix Cluster"(w177) -> ()
              }
            }
            n127 = local write "Timing"(w160) -> ()
          }
          event "Start\nWater 2": Value Change {
            n128 = event-data() -> ("NewVal"=w213:dbl)  [unwired: 1 in, 5 out]
            n129 = local read "Mix Cluster"() -> (w216:T2)
            n130 = for {
              tunnel: w216 -> [w220] mode=indexing
              tunnel: [w217] -> w215 mode=indexing
              n131 = Unbundle By Name(w220) -> ("Odor Time"=w219:dbl, "Water Time"=w218:dbl)
              n132 = Add(x=w219, y=w218) -> (x+y=w217:dbl)
            }
            n133 = local write "Start Water"(w213) -> ()
            n134 = Add Array Elements(numeric array=w215) -> (sum=w214:dbl)
            n135 = Add(x=w214, y=w213) -> (x+y=w212:dbl)
            n136 = local write "Experiment Time (Sec)"(w212) -> ()
          }
          event "Start Water": Value Change {
            n137 = event-data() -> ("NewVal"=w221:dbl)  [unwired: 1 in, 5 out]
            n138 = local read "Mix Cluster"() -> (w222:T2)
            n139 = for {
              tunnel: w222 -> [w229] mode=indexing
              tunnel: [w226] -> w223 mode=indexing
              n140 = Unbundle By Name(w229) -> ("Odor Time"=w228:dbl, "Water Time"=w227:dbl)
              n141 = Add(x=w228, y=w227) -> (x+y=w226:dbl)
            }
            n142 = local write "Start\nWater 2"(w221) -> ()
            n143 = Add Array Elements(numeric array=w223) -> (sum=w224:dbl)
            n144 = Add(x=w224, y=w221) -> (x+y=w225:dbl)
            n145 = local write "Experiment Time (Sec)"(w225) -> ()
          }
          event "Use Control": Value Change {
            n146 = event-data() -> ("NewVal"=w230:bool)  [unwired: 1 in, 5 out]
            n147 = disable-structure shown="Disabled" {
              disable-tunnel: w230 -> [w231 _]
              frame Disabled {
                n148 = control-ref of="Ctr Odor Valve"() -> (w238:refnum<vi>)
                n149 = control-ref of="Valves"() -> (w236:refnum<vi>)
                n150 = control-ref of="Pressure Group"() -> (w233:refnum<vi>)
                n151 = control-ref of="Odor"() -> (w234:refnum<vi>)
                n152 = control-ref of="Ring"() -> (w235:refnum<vi>)
                n153 = control-ref of="Ctr Pressure\n Group"() -> (w240:refnum<vi>)
                n154 = control-ref of="Mix Water Valve"() -> (w239:refnum<vi>)
                n155 = case shown="True" w231 {
                  frame False {
                    (unwired) 16
                  }
                  frame True {
                    (unwired) 13
                  }
                }
                n156 = control-ref of="Water Mix \nPressure Group"() -> (w241:refnum<vi>)
                n157 = Build Array(w236, w235, w234, w233) -> (w232:refnum<vi>[])
                n158 = Build Array(w241, w240, w239, w238) -> (w237:refnum<vi>[])  [unwired: 1 in]
                n159 = for {
                  tunnel: w232 -> [_] mode=indexing
                }
                n160 = for {
                  tunnel: w237 -> [w243] mode=indexing
                  tunnel: w231 -> [w242]
                  n161 = property class="Num"(reference=w243, "Visible"=w242) -> ()  [unwired: 1 in, 2 out]
                }
                n162 = control-ref of="Odor \nLevel"() -> ()  [unwired: 1 out]
                n163 = control-ref of="Refill!"() -> ()  [unwired: 1 out]
              }
              frame Enabled {
              }
            }
          }
          event "Total Flow Setpoint", "Total Odor Flow": Value Change {
            n164 = event-data() -> ()  [unwired: 1 in, 6 out]
            n165 = local read "Total Odor Flow"() -> (w245:dbl)
            n166 = local read "Total Flow Setpoint"() -> (w244:dbl)
            n167 = global write "ValveGlobals.vi" "Total Flow Setpoint"(w244) -> ()
            n168 = global write "ValveGlobals.vi" "Total Odor Flow"(w245) -> ()
          }
          event "Refill!": Value Change {
            n169 = event-data() -> ("NewVal"=w246:bool[])  [unwired: 1 in, 5 out]
            n170 = flat-sequence {
              tunnel: w247 -> [w249]
              tunnel: w246 -> [w248]
              frame #0 {
                n171 = Send Notification(notification=w248, notifier=w249) -> ()  [unwired: 1 in, 2 out]
              }
              frame #1 {
                n172 = local write "Refill!"(bool[] [FALSE, FALSE, FALSE, FALSE, FALSE, FALSE, FALSE, FALSE, FALSE, FALSE, FALSE] ("Refill!")) -> ()
              }
            }
          }
          event "Begin Experiment": Value Change {
            w284 = "_run" ("string")
            n173 = event-data() -> ()  [unwired: 1 in, 6 out]
            n174 = local read "Start Water"() -> (w293:dbl)
            n175 = Build Array(w293) -> (w292:dbl[])
            n176 = local read "Mix Cluster"() -> (w279:T2)
            n177 = local read "Log Folder"() -> (w258:path)
            n178 = for {
              shift-right: [w301] -> w288
              shift-left: w292 -> [w305]
              tunnel: w279 -> [w304] mode=indexing
              tunnel: [w298] -> w264 mode=concatenating
              n179 = Unbundle By Name(w304) -> ("Odor Time"=w303:dbl, "Water Time"=w302:dbl, "Mixture List"=w299:string)
              n180 = Build Array (concatenate)(w305, w303, w302) -> (w301:dbl[])
              n181 = Build Array(w299, "water" ("element")) -> (w298:string[])
            }
            n182 = local read "Set Pressure Cluster"() -> (w253:T1)
            n183 = local read "Possible Water Mix Ratios"() -> (w277:dbl[])
            n184 = Unbundle By Name(w253) -> ("Control Pressure"=w252:dbl)
            n185 = local read "Mix Water Pressure Channel"() -> (w276:u16)
            n186 = Number To Decimal String(number="_run") -> (decimal integer string=w283:string)  [unwired: 1 in]
            n187 = local read "Mix Sequence Array"() -> (w270:bool[][])
            n188 = local read "Default Pressures"() -> (w254:dbl[])
            n189 = local read "Mix Water Valve"() -> (w251:u16)
            n190 = local read "Calibration Refs"() -> (w297:T3)
            n191 = local read "Pressure Group"() -> (w278:enum16{"1", "2", "3", "4"}[])
            n192 = local read "Ctr Odor Valve"() -> (w295:u16)
            n193 = Concatenate Strings("Log File Name", w284, w283, ".h5" ("string")) -> (w281:string)
            n194 = Concatenate Strings("log_" ("string"), "Log File Name", w284, w283) -> (w266:string)
            n195 = Build Array (concatenate)("water" ("element"), w264) -> (w262:string[])
            n196 = local read "Concentration Strings"() -> (w272:string[])
            n197 = local read "Ctr Pressure\n Group"() -> (w274:u8)
            n198 = local read "Odor Strings"() -> (w271:string[])
            n199 = call "Check If Calibration Data Exist_MultiMix.vi"("Set Pressure Cluster"=w253, "Water Mix Pressure Group"=w276, "Mix Sequence Array"=w270, "Water Mix Valve"=w251, "Possible Water Mix Ratios"=w277, "Pressure Group"=w278, "Calibration Refs"=w297) -> ("Calibration Data Exists?"=w296:bool, "Psequence"=w275:dbl[][])  [unwired: 3 in]
            n200 = Build Path(base path=w258, name or relative path=w281) -> (appended path=w280:path)
            n201 = local read "Valves"() -> (w273:u16[])
            n202 = Concatenate Strings(w266, ".h5" ("string")) -> (w267:string)
            n203 = Concatenate Strings(w266, ".txt" ("string")) -> (w268:string)
            n204 = call "AddControlPressure2Psequence.vi"("Control Pressure"=w252, "Ctr Pressure Channel"=w274, "Psequence"=w275) -> ("Psequence Out"=w256:dbl[][])  [unwired: 8 in]
            n205 = call "fill_in_missing_pressures.vi"("Default Pressures"=w254, "Pressure Sequence"=w256) -> ("Pressure Sequence Out"=w255:dbl[][])  [unwired: 9 in]
            n206 = call "GenerateLogFile.vi"("Mixture Strings"=w262, "Sequence Time"=w288, "Mix Sequence Array"=w270, "Concentration Names"=w272, "Odor Names"=w271) -> ("Log Cluster"=w261:T15, "Text Log Data"=w286:string[][])  [unwired: 5 in]
            n207 = Build Path(base path=w258, name or relative path=w268) -> (appended path=w287:path)
            n208 = Build Path(base path=w258, name or relative path=w267) -> (appended path=w260:path)
            n209 = call "GenerateValveSequenceMultiMix.vi"("Mix Water Valve"=w251, "Ctr Water Valve"="Ctr Water Valve", "Ctr Odor Valve"=w295, "Valves"=w273, "Mix Sequence Array"=w270) -> ("Valve Sequence Data"=w294:T16)  [unwired: 6 in]
            n210 = case shown="True" w296 {
              tunnel: w294 -> [_ w317]
              tunnel: w288 -> [_ w319]
              tunnel: w255 -> [_ w318]
              tunnel: w291 -> [_ w320]
              tunnel: "_run" -> [_ w315]
              tunnel: w287 -> [_ w312]
              tunnel: w286 -> [_ w314]
              tunnel: "Sync Camera Acquisition" -> [_ w313]
              tunnel: w280 -> [_ w311]
              tunnel: w262 -> [_ w310]
              tunnel: w261 -> [_ w309]
              tunnel: w260 -> [_ w308]
              frame False {
                n211 = One Button Dialog(message="Calibration Required First!") -> ()  [unwired: 1 in, 1 out]
              }
              frame True {
                n212 = call "run_experiment_multi_mix.vi"("Sync Camera Acquisition"=w313, "Log File Name"=w311, "Pressure Sequence"=w318, "Valve Sequence Data"=w317, "mixture sequence array"=w310, "Time Sequence"=w319, "MFCS_EZ"=w320) -> ("Aborted?"=w316:bool, "Flow Data Out"=w307:T17)  [unwired: 3 in]
                n213 = case shown="False" w316 {
                  tunnel: w315 -> [w327 _]
                  tunnel: w312 -> [w325 _]
                  tunnel: w314 -> [w324 _]
                  tunnel: w309 -> [w323 _]
                  tunnel: w308 -> [w322 _]
                  tunnel: w307 -> [w321 _]
                  frame False {
                    n214 = call-poly <vilib>:"Write Delimited Spreadsheet.vi"("file path (dialog if empty)"=w325, "2D data"=w324) -> ()  [unwired: 12 in, 2 out]
                    n215 = call "make_log_file_H5.vi"("Path"=w322, "Log Cluster"=w323, "Flow Data"=w321) -> ()  [unwired: 8 in]
                    n216 = Increment(x=w327) -> (x+1=w326:i16)
                    n217 = local write "_run"(w326) -> ()
                    "Saved Log File Name" <- w322
                  }
                  frame True {
                  }
                }
              }
            }
          }
          event "Odor Inf Path": Value Change {
            n218 = event-data() -> ("NewVal"=w332:path)  [unwired: 1 in, 5 out]
            n219 = call-poly <vilib>:"Read Delimited Spreadsheet.vi"("file path (dialog if empty)"=w332) -> ("error out"=w334:errorcluster)  [unwired: 9 in, 5 out]
            n220 = Unbundle By Name(w334) -> ("code"=w333:i32)
            n221 = case shown="0, Default" w333 {
              tunnel: w332 -> [w337 w342]
              tunnel: [w336 w339] -> w331
              tunnel: [w335 w338] -> w330
              frame 0, Default {
                n222 = call "LoadOdorInf.vi"("file path (dialog if empty)"=w337) -> ("Concentration"=w335:string[], "Odor"=w336:string[])  [unwired: 9 in]
              }
              frame 7 {
                n223 = call-poly <vilib>:"Write Delimited Spreadsheet.vi"("file path (dialog if empty)"=w342, "2D data"=string[][] []) -> ("new file path (Not A Path if cancelled)"=w340:path)  [unwired: 12 in, 1 out]
                n224 = call "LoadOdorInf.vi"("file path (dialog if empty)"=w340) -> ("Concentration"=w338:string[], "Odor"=w339:string[])  [unwired: 9 in]
              }
            }
            n225 = control-ref of="Concentration"() -> (w329:refnum<vi>)
            n226 = control-ref of="Odor"() -> (w328:refnum<vi>)
            n227 = call "PopulateRingArrays.vi"("array"=w330, "Array Reference"=w329) -> ()  [unwired: 8 in, 2 out]
            n228 = call "PopulateRingArrays.vi"("array"=w331, "Array Reference"=w328) -> ()  [unwired: 8 in, 2 out]
          }
          event "Save Odor Inf File": Value Change {
            n229 = event-data() -> ()  [unwired: 1 in, 6 out]
            n230 = control-ref of="Concentration"() -> (w345:refnum<vi>)
            n231 = control-ref of="Odor"() -> (w344:refnum<vi>)
            n232 = local read "Odor Inf Path"() -> (w347:path)
            n233 = property class="Ring (strict)"(reference=w345) -> ("Strings []"=w346:string[])  [unwired: 1 in, 2 out]
            n234 = property class="Ring (strict)"(reference=w344) -> ("Strings []"=w343:string[])  [unwired: 1 in, 2 out]
            n235 = call "SaveOdorInf.vi"("Path"=w347, "Concentrations"=w346, "Odors"=w343) -> ()  [unwired: 9 in]
          }
          event "Set to default pressure", "Set to default pressure 2": Value Change {
            n236 = event-data() -> ()  [unwired: 1 in, 6 out]
            n237 = local read "Default Pressures"() -> (w349:dbl[])
            n238 = local write "Manual Set Pressures"(w349) -> ()
            n239 = for {
              tunnel: w348 -> [w353]
              tunnel: w349 -> [w352] mode=indexing
              i -> [w351]
              n240 = Increment(x=w351) -> (x+1=w350:i32)
              n241 = call-poly <userlib>:"MFCS Write Channel Pressure.vi"("MFCS_EZ"=w353, "Channel Number (default=1)"=w350, "Pressure (mBar)"=w352) -> ()  [unwired: 11 in, 2 out]
            }
          }
          event "Close All Valves": Value Change {
            n242 = event-data() -> ()  [unwired: 1 in, 6 out]
            n243 = call "close_all_channels.vi"() -> ()  [unwired: 12 in]
          }
          event "Zero Pressure 2", "Zero Pressure": Value Change {
            n244 = event-data() -> ()  [unwired: 1 in, 6 out]
            n245 = for {
              N: 4 -> [_]
              tunnel: w354 -> [w356]
              i -> [w359]
              n246 = Increment(x=w359) -> (x+1=w358:i32)
              n247 = call-poly <userlib>:"MFCS Write Channel Pressure.vi"("MFCS_EZ"=w356, "Channel Number (default=1)"=w358, "Pressure (mBar)"=0.0) -> ()  [unwired: 11 in, 2 out]
            }
          }
          event "Base Folder": Value Change {
            n248 = event-data() -> ("NewVal"=w361:path)  [unwired: 1 in, 5 out]
            n249 = call "CreateLogFolder.vi"("Base Folder"=w361) -> ("Path Out"=w360:path)  [unwired: 9 in, 1 out]
            n250 = local write "Log Folder"(w360) -> ()
          }
          event "New Animal": Value Change {
            w364 = i16 100 ("x")
            n251 = event-data() -> ()  [unwired: 1 in, 6 out]
            n252 = local read "_run"() -> (w365:i16)
            n253 = call "Round to nearest.vi"("Round to nearest"=w364, "Number"=w365) -> ("Rounded"=w363:dbl)  [unwired: 9 in]
            n254 = Add(x=w364, y=w363) -> (x+y=w366:dbl)
            n255 = Increment(x=w366) -> (x+1=w362:dbl)
            n256 = local write "_run"(w362) -> ()
          }
          event "Manual Set Pressures": Value Change {
            n257 = event-data() -> ("NewVal"=w367:dbl[])  [unwired: 1 in, 5 out]
            n258 = for {
              tunnel: w368 -> [w372]
              tunnel: w367 -> [w371] mode=indexing
              i -> [w370]
              n259 = Increment(x=w370) -> (x+1=w369:i32)
              n260 = call-poly <userlib>:"MFCS Write Channel Pressure.vi"("MFCS_EZ"=w372, "Channel Number (default=1)"=w369, "Pressure (mBar)"=w371) -> ()  [unwired: 11 in, 2 out]
            }
          }
          event "Odor", "Concentration": Value Change {
            n261 = event-data() -> ("CtlRef"=w374:refnum<vi>, "OldVal"=w373:u16[], "NewVal"=w375:u16[])  [unwired: 1 in, 3 out]
            n262 = flat-sequence {
              tunnel: w375 -> [w384]
              tunnel: w374 -> [w382]
              tunnel: w373 -> [w376]
              frame #0 {
                n263 = call "GetRingRef.vi"("Array Reference"=w382) -> ("Ring Reference"=w385:refnum<vi>)  [unwired: 9 in, 1 out]
                n264 = property class="Ring"(reference=w385) -> ("NumItems"=w383:u32, "Strings []"=w381:string[])  [unwired: 1 in, 2 out]
                n265 = Array Size(array=w381) -> (size(s)=w380:i32)
                n266 = Decrement(x=w380) -> (x-1=w377:i32)
                n267 = Delete From Array(array=w381, length=1, index=w377) -> (array with subset deleted=w378:string[])  [unwired: 1 out]
                n268 = for {
                  tunnel: w384 -> [w392] mode=indexing
                  tunnel: w383 -> [w391]
                  tunnel: w382 -> [w389]
                  tunnel: w378 -> [w388]
                  tunnel: w376 -> [w386]
                  n269 = Increment(x=w392) -> (x+1=w387:u16)
                  n270 = Equal?(x=w391, y=w387) -> (x = y?=w390:bool)
                  n271 = case shown="True" w390 {
                    tunnel: w389 -> [_ w399]
                    tunnel: w388 -> [_ w400]
                    tunnel: w386 -> [_ w398]
                    frame False {
                    }
                    frame True {
                      n272 = call "AddNewOdorsConc.vi"() -> ("To Add Out"=w396:string[])  [unwired: 10 in]
                      n273 = Build Array (concatenate)(w400, w396) -> (w397:string[])
                      n274 = Array Size(array=w396) -> (size(s)=w395:i32)
                      n275 = Equal?(x=w395, y=0 ("size(s)")) -> (x = y?=w393:bool)
                      n276 = case shown="False" w393 {
                        tunnel: w399 -> [w403 w408]
                        tunnel: w398 -> [_ w407]
                        tunnel: w397 -> [w402 _]
                        frame False {
                          n277 = call "PopulateRingArrays.vi"("array"=w402, "Array Reference"=w403) -> ()  [unwired: 8 in, 2 out]
                          n278 = case shown="True" "Append Changes To Odor Inf File" {
                            frame False {
                            }
                            frame True {
                              n279 = local read "Odor Inf Path"() -> (w404:path)
                              n280 = control-ref of="Concentration"() -> (w406:refnum<vi>)
                              n281 = control-ref of="Odor"() -> (w405:refnum<vi>)
                              n282 = call "UpdateOdorConcInf.vi"("Path"=w404, "Concentration Ref"=w406, "Odor Ref"=w405) -> ()  [unwired: 9 in]
                            }
                          }
                        }
                        frame True {
                          n283 = property class="Arr (strict)"(reference=w408, "Value"=w407) -> ()  [unwired: 1 in, 2 out]
                        }
                      }
                    }
                  }
                }
              }
              frame #1 {
                n284 = local read "Concentration"() -> (w412:u16[])
                n285 = control-ref of="Concentration"() -> (w414:refnum<vi>)
                n286 = local read "Odor"() -> (w413:u16[])
                n287 = control-ref of="Odor"() -> (w415:refnum<vi>)
                n288 = call "MakeOdorConcStrings.vi"(8:"Concentration"=w412, 9:"Odor"=w413, 10:"Concentration"=w414, 11:"Odor"=w415) -> ("Concentration Strings"=w411:string[], "Odor Strings"=w410:string[])  [unwired: 6 in]
                n289 = for {
                  tunnel: w411 -> [w419] mode=indexing
                  tunnel: w410 -> [w418] mode=indexing
                  tunnel: [w416] -> w409 mode=indexing
                  n290 = call <vilib>:"Space Constant.vi"() -> ("String"=w417:string)
                  n291 = Concatenate Strings(w419, w417, w418) -> (w416:string)
                }
                "Odor List" <- w409
                n292 = local write "Odor Strings"(w410) -> ()
                n293 = local write "Concentration Strings"(w411) -> ()
              }
            }
          }
          event "Valves": Value Change {
            # "greater than 0 means there are duplicates"
            n294 = event-data() -> ("NewVal"=w422:u16[])  [unwired: 1 in, 5 out]
            n295 = local read "Ctr Odor Valve"() -> (w420:u16)
            n296 = global write "ValveGlobals.vi" "Ctr Odor Valve"(w420) -> ()
            n297 = global write "ValveGlobals.vi" "Valves Used"("Valves") -> ()
            n298 = call-poly <userlib>:"Remove Duplicates from 1D Array__ogtk.vi"("Input Array"=w422) -> ("indices of removed elements"=w426:i32[])  [unwired: 1 out]
            n299 = Array Size(array=w426) -> (size(s)=w424:i32)
            n300 = Greater?(x=w424, y=0 ("x")) -> (0:w423:bool)
            "Duplicates!" <- w423
            n301 = property on="Duplicates!" class="Bool (strict)"("Blinking"=w423, "Visible"=w423) -> ()  [unwired: 2 in, 2 out]
          }
          event "Number of Periods": Value Change {
            n302 = event-data() -> ()  [unwired: 1 in, 6 out]
            n303 = local read "Master Mix Sequence Array"() -> (w454:bool[][])
            n304 = local read "Mix Sequence Control"() -> (w437:bool[][])
            n305 = local read "Mix Sequence Array"() -> (w458:bool[][])
            n306 = control-ref of="Timing"() -> (w430:refnum<vi>)
            n307 = control-ref of="Mix Sequence Array"() -> (w457:refnum<vi>)
            n308 = case shown="1, Default" "Number of Periods" {
              selector: "Number of Periods" -> [w474 _]
              tunnel: [w474 w475] -> w431
              frame 1, Default {
              }
              frame 0 {
                w475 = 1
                n309 = local write "Number of Periods"(w475) -> ()
              }
            }
            n310 = control-ref of="Mix Sequence Control"() -> (w436:refnum<vi>)
            n311 = Transpose 2D Array(2D array=w458) -> (transposed array=w452:bool[][])
            n312 = Transpose 2D Array(2D array=w454) -> (transposed array=w453:bool[][])
            n313 = for {
              tunnel: w452 -> [w500] mode=indexing
              tunnel: w453 -> [w492] mode=indexing
              tunnel: w457 -> [w499]
              tunnel: w431 -> [w488]
              tunnel: [w496] -> w455 mode=indexing
              tunnel: [w495] -> w456 mode=indexing
              tunnel: w437 -> [w490] mode=indexing
              tunnel: w436 -> [w493]
              tunnel: [w489] -> w435 mode=indexing
              tunnel: [w486] -> w429
              w486 = u16 0 ("Max Visible Size")
              n314 = call "MakeArrayRightSize.vi"("Row or Column"=enum16{"Rows", "Columns"}."Columns", "Max Visible Size"=w486, "Size"=w488, "Master Array In"=w492, "Array"=w490, "reference"=w493) -> ("Array Out"=w491:variant[])  [unwired: 4 in, 1 out]
              n315 = call "MakeArrayRightSize.vi"("Max Visible Size"=u16 0, "Size"=w488, "Master Array In"=w492, "Array"=w500, "reference"=w499) -> ("Array Out"=w497:variant[], "Master Array Out"=w498:variant[])  [unwired: 5 in]
              n316 = Variant To Data(type=w492, Variant=w498) -> (data=w495:bool[])  [unwired: 1 in, 1 out]
              n317 = Variant To Data(type=w492, Variant=w497) -> (data=w496:bool[])  [unwired: 1 in, 1 out]
              n318 = Variant To Data(type=w490, Variant=w491) -> (data=w489:bool[])  [unwired: 1 in, 1 out]
            }
            n319 = for {
              tunnel: "Timing" -> [w464] mode=indexing
              tunnel: "Master Timing" -> [w473] mode=indexing
              tunnel: w431 -> [w472]
              tunnel: w430 -> [w470]
              tunnel: w429 -> [w469]
              tunnel: [w466] -> w428 mode=indexing
              tunnel: [w465] -> w427 mode=indexing
              n320 = call "MakeArrayRightSize.vi"("Row or Column"=enum16{"Rows", "Columns"}."Columns", "Max Visible Size"=w469, "Size"=w472, "Master Array In"=w473, "Array"=w464, "reference"=w470) -> ("Array Out"=w468:variant[], "Master Array Out"=w467:variant[])  [unwired: 4 in]
              n321 = Variant To Data(type=w464, Variant=w467) -> (data=w466:dbl[])  [unwired: 1 in, 1 out]
              n322 = Variant To Data(type=w464, Variant=w468) -> (data=w465:dbl[])  [unwired: 1 in, 1 out]
            }
            n323 = local read "Mix Cluster"() -> (w443:T2)
            n324 = control-ref of="Mix Cluster"() -> (w449:refnum<vi>)
            n325 = Transpose 2D Array(2D array=w456) -> (transposed array=w451:bool[][])
            n326 = Transpose 2D Array(2D array=w455) -> (transposed array=w450:bool[][])
            n327 = local write "Master Timing"(w428) -> ()
            n328 = local write "Timing"(w427) -> ()
            n329 = local write "Mix Sequence Control"(w435) -> ()
            n330 = local write "Master Mix Sequence Array"(w451) -> ()
            n331 = local write "Mix Sequence Array"(w450) -> ()
            n332 = for {
              tunnel: w450 -> [w485] mode=indexing
              tunnel: [w482] -> w445 mode=indexing
              n333 = local read "Concentration Strings"() -> (w483:string[])
              n334 = local read "Odor Strings"() -> (w484:string[])
              n335 = call "CreateMixtureString.vi"("Odor Mixtures"=w485, "Concentrations"=w483, "Odors"=w484) -> ("Odor Mixture String"=w482:string)  [unwired: 8 in]
            }
            n336 = for {
              tunnel: w443 -> [w478] mode=indexing
              tunnel: [w477] -> w442 mode=indexing
              tunnel: [w476] -> w441 mode=indexing
              n337 = Unbundle By Name(w478) -> ("Odor Time"=w477:dbl, "Water Time"=w476:dbl)
            }
            n338 = call "MakeArrayRightSize.vi"("Max Visible Size"=u16 7, "Size"=w431, "Master Array In"="Master Mix Cluster", "Array"=w443, "reference"=w449) -> ("Array Out"=w448:variant[], "Master Array Out"=w447:variant[])  [unwired: 5 in]
            n339 = Variant To Data(type=w443, Variant=w448) -> (data=w440:T2)  [unwired: 1 in, 1 out]
            n340 = Variant To Data(type=w443, Variant=w447) -> (data=w446:T2)  [unwired: 1 in, 1 out]
            n341 = local write "Master Mix Cluster"(w446) -> ()
            n342 = Add Array Elements(numeric array=w442) -> (sum=w463:dbl)
            n343 = Add Array Elements(numeric array=w441) -> (sum=w462:dbl)
            n344 = Add(x=w463, y=w462) -> (x+y=w461:dbl)
            n345 = Add(x="Start Water", y=w461) -> (x+y=→"Experiment Time (Sec)":dbl)
            n346 = for {
              tunnel: w440 -> [w481] mode=indexing
              tunnel: w445 -> [w480] mode=indexing
              tunnel: [w479] -> w444 mode=indexing
              n347 = Bundle By Name(cluster=w481, "Mixture List"=w480) -> (w479:T14)
            }
            n348 = local write "Mix Cluster"(w444) -> ()
          }
          event "Timing": Value Change {
            n349 = event-data() -> ("NewVal"=w511:dbl[][])  [unwired: 1 in, 5 out]
            n350 = local read "Mix Cluster"() -> (w508:T2)
            n351 = Index Array(array=w511, index (row) #1=0 ("index (row)"), index (row) #2=1 ("index (row)")) -> (element #1=w506:dbl[], element #2=w505:dbl[])  [unwired: 2 in]
            n352 = for {
              tunnel: w508 -> [w516] mode=indexing
              tunnel: [w515] -> w507 mode=indexing
              tunnel: w506 -> [w514] mode=indexing
              tunnel: w505 -> [w513] mode=indexing
              tunnel: [w512] -> w504 mode=indexing
              n353 = Bundle By Name(cluster=w516, "Odor Time"=w514, "Water Time"=w513) -> (w515:T14)
              n354 = Add(x=w514, y=w513) -> (x+y=w512:dbl)
            }
            n355 = local read "Start Water"() -> (w502:dbl)
            n356 = local write "Mix Cluster"(w507) -> ()
            n357 = Add Array Elements(numeric array=w504) -> (sum=w503:dbl)
            n358 = Add(x=w502, y=w503) -> (x+y=w501:dbl)
            n359 = local write "Experiment Time (Sec)"(w501) -> ()
          }
          event "Save Button", "Load Button": Value Change {
            n360 = event-data() -> ("CtlRef"=w532:refnum<vi>)  [unwired: 1 in, 5 out]
            n361 = Current VI's Path() -> (path=w524:path)
            n362 = Strip Path(path=w524) -> (stripped path=w522:path)  [unwired: 1 out]
            n363 = Strip Path(path=w522) -> (stripped path=w521:path)  [unwired: 1 out]
            n364 = local read "Max Number of\nOdors in Mixture"() -> (w538:u16)
            n365 = Build Path(base path=w521, name or relative path="OdorInf") -> (appended path=w529:path)
            n366 = local read "Mix Sequence Array"() -> (w541:bool[][])
            n367 = local read "Set Pressure Cluster"() -> (w536:T1)
            n368 = local read "Default Pressures"() -> (w537:dbl[])
            n369 = local read "Number of Periods"() -> (w520:u16)
            n370 = local read "Calibration Refs"() -> (w534:T3)
            n371 = local read "Pressure Group"() -> (w542:enum16{"1", "2", "3", "4"}[])
            n372 = local read "Concentration"() -> (w544:u16[])
            n373 = local read "Base Dilution"() -> (w539:dbl)
            n374 = local read "Start Water"() -> (w540:dbl)
            n375 = Build Path(base path=w529, name or relative path="Data") -> (appended path=w527:path)
            n376 = local read "Mix Cluster"() -> (w535:T2)
            n377 = local read "Valves"() -> (w545:u16[])
            n378 = local read "Odor"() -> (w543:u16[])
            n379 = Build Path(base path=w527, name or relative path="GUIConfig") -> (appended path=w525:path)
            n380 = property class="Bool"(reference=w532) -> ("Label.Text"=w531:string)  [unwired: 1 in, 2 out]
            n381 = Bundle("Valves"=w545, "Concentration"=w544, "Odor"=w543, "Pressure Group"=w542, "Mix Sequence Array"=w541, "Start Water"=w540, "Base Dilution"=w539, "Max Number of\nOdors in Mixture"=w538, "Default Pressures"=w537, "Set Pressure Cluster"=w536, "Mix Cluster"=w535, "Calibration Refs"=w534, "Number of Periods"=w520) -> (w533:T18)  [unwired: 1 in]
            n382 = case shown="\"Load Button\", Default" w531 {
              tunnel: w533 -> [w554 w601]
              tunnel: w525 -> [w556 w594]
              tunnel: [w549 w590] -> w523
              tunnel: [w547 w589] -> w519
              tunnel: "load unsuccessful" ("load status") -> [w546 _]
              tunnel: "save unsuccessful" ("load status") -> [_ w588]
              frame "Load Button", Default {
                n383 = call "File Dialog2"("start path"=w556) -> ("selected path"=w555:path, "exists"=w552:bool, "cancelled"=w553:bool, "error out"=w548:errorcluster)  [unwired: 11 in]
                n384 = Not(x=w552) -> (.not. x?=w551:bool)
                n385 = Or(x=w551, y=w553) -> (x .or. y?=w550:bool)
                n386 = case shown="False" w550 {
                  selector: w550 -> [_ w587]
                  tunnel: w555 -> [w567 _]
                  tunnel: w554 -> [w565 _]
                  tunnel: [w561 w587] -> w549
                  tunnel: w548 -> [w560 _]
                  tunnel: [w558 w586] -> w547
                  tunnel: w546 -> [w557 w586]
                  frame False {
                    n387 = call-poly <vilib>:"Read From XML File.vi"("error in (no error)"=w560, "XML File Path"=w567) -> ("error out"=w563:errorcluster, "XML Elements"=w566:string, "XML File Path(duplicate)"=w559:path)  [unwired: 7 in]
                    n388 = Unflatten From XML(xml string=w566, type=w565, error in (no error)=w563) -> (value=w564:T18, error out=w562:errorcluster)
                    n389 = Unbundle By Name(w562) -> ("status"=w561:bool)
                    n390 = case shown="False" w561 {
                      tunnel: w564 -> [w584 _]
                      tunnel: [w569 w585] -> w558
                      tunnel: w559 -> [w570 _]
                      tunnel: w557 -> [_ w585]
                      frame False {
                        n391 = Unbundle By Name(w584) -> ("Valves"=w576:u16[], "Concentration"=w575:u16[], "Odor"=w574:u16[], "Pressure Group"=w573:enum16{"1", "2", "3", "4"}[], "Mix Sequence Array"=w577:bool[][], "Start Water"=w579:dbl, "Base Dilution"=w578:dbl, "Max Number of\nOdors in Mixture"=w580:u16, "Default Pressures"=w581:dbl[], "Set Pressure Cluster"=w568:T1, "Mix Cluster"=w582:T2, "Calibration Refs"=w583:T3, "Number of Periods"=w571:u16)
                        n392 = control-ref of="Number of Periods"() -> (w572:refnum<vi>)
                        n393 = local write "Valves"(w576) -> ()
                        n394 = local write "Odor"(w574) -> ()
                        n395 = local write "Set Pressure Cluster"(w568) -> ()
                        n396 = local write "Mix Sequence Array"(w577) -> ()
                        n397 = local write "Start Water"(w579) -> ()
                        n398 = local write "Base Dilution"(w578) -> ()
                        n399 = local write "Max Number of\nOdors in Mixture"(w580) -> ()
                        n400 = local write "Default Pressures"(w581) -> ()
                        n401 = local write "Concentration"(w575) -> ()
                        n402 = local write "Pressure Group"(w573) -> ()
                        n403 = local write "Mix Cluster"(w582) -> ()
                        n404 = local write "Calibration Refs"(w583) -> ()
                        n405 = property class="DigNum (strict)"(reference=w572, "Val(Sgnl)"=w571) -> ()  [unwired: 1 in, 2 out]
                        n406 = Strip Path(path=w570) -> (name=w569:string)  [unwired: 1 out]
                      }
                      frame True {
                      }
                    }
                  }
                  frame True {
                  }
                }
              }
              frame "Save Button" {
                n407 = Flatten To XML(anything=w601) -> (xml string=w602:string)
                n408 = Get Date/Time In Seconds() -> (seconds since 1Jan1904=w596:timestamp)
                n409 = Format Date/Time String(time format string (%c)="%Y%m%d", seconds (now)=w596) -> (date/time string=w598:string)  [unwired: 1 in]
                n410 = Concatenate Strings(w598, "_config.xml" ("string")) -> (w600:string)
                n411 = call "File Dialog"("start path"=w594, "default name"=w600) -> ("selected path"=w595:path, "cancelled"=w593:bool, "error out"=w592:errorcluster)  [unwired: 10 in, 1 out]
                n412 = case shown="False" w593 {
                  tunnel: w602 -> [w608 _]
                  tunnel: w595 -> [w607 _]
                  tunnel: w592 -> [w606 w610]
                  tunnel: [w605 w610] -> w591
                  tunnel: w588 -> [_ w609]
                  tunnel: [w603 w609] -> w589
                  frame False {
                    n413 = call-poly <vilib>:"Write to XML File.vi"("error in (no error)"=w606, "XML Input"=w608, "XML File Path"=w607) -> ("error out"=w605:errorcluster, "XML File Path(duplicate)"=w604:path)  [unwired: 6 in, 1 out]
                    n414 = Strip Path(path=w604) -> (name=w603:string)  [unwired: 1 out]
                  }
                  frame True {
                  }
                }
                n415 = Unbundle By Name(w591) -> ("status"=w590:bool)
              }
            }
            "status" <- w523
            "load status" <- w519
          }
          event "Max Number of\nOdors in Mixture": Value Change {
            n416 = event-data() -> ()  [unwired: 1 in, 6 out]
            n417 = Reciprocal(x="Max Number of\nOdors in Mixture") -> (1/x=→"Base Dilution":dbl)
          }
          event "Reset All Calibrations": Value Change {
            n418 = event-data() -> ()  [unwired: 1 in, 6 out]
            n419 = Two Button Dialog(message="Are you sure? Calibration will be required before any experiments.") -> (T button?=w613:bool)  [unwired: 2 in]
            n420 = case shown="True" w613 {
              frame False {
              }
              frame True {
                n421 = Bundle By Name(cluster=T3 {"Pressure Controller List"=[3, 3, 3], "Ratio List"=[0.6, 0.6, 0.5], "Valve List"=[0, 1, 1]} ("Calibration Refs"), "Pressure Controller List"=u8[] [], "Ratio List"=dbl[] [], "Valve List"=u16[] []) -> (w615:T3)
                n422 = local write "Calibration Refs"(w615) -> ()
              }
            }
          }
          event "stop": Value Change {
            n423 = event-data() -> ()  [unwired: 1 in, 6 out]
            n424 = call-poly <userlib>:"MFCS Close.vi"("MFCS_EZ"=w624) -> ()  [unwired: 14 in, 1 out]
            n425 = control-ref of="This VI"() -> (w622:refnum<vi>)
            n426 = call <vilib>:"Save State As Default.vi"("Target VI"=w622) -> ()  [unwired: 9 in, 2 out]
            n427 = Send Notification(notification="quit", notifier=w621) -> ()  [unwired: 1 in, 2 out]
          }
        }
      }
    }
  }
